vi "Attenuator Flatten Test Parameters.vi"(7 "Test Configuration (\"\")":string, 9 "error in (no error)":errorcluster, 10 "Parameter Variant":variant) -> (1 "error out":errorcluster, 2 "Parameter String":string)   [LabVIEW 2011]
uses:
  TypeDefs/Attenuator Test Parameters.ctl
  TypeDefs/Attenuator Stimulus Parameters.ctl
  TypeDefs/Attenuator ATT Stimulus.ctl
  TypeDefs/Attenuator VNA Stimulus.ctl
  S Parameter/TypeDefs/SP Frequency Units.ctl
  TypeDefs/Attenuator VNA Calibration State.ctl
  TypeDefs/Attenuator Measurement Cluster.ctl
  TypeDefs/Attenuator Limit.ctl
  TypeDefs/Attenuator Calibration State.ctl
  Attenuator Version.vi
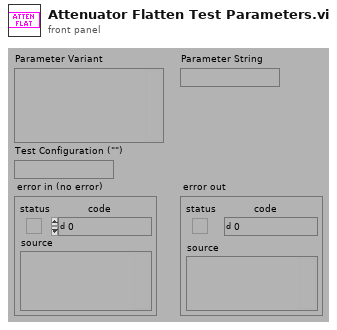
[diagram p1: front panel]
types:
  T1 = typedef "Attenuator Test Parameters.ctl" = cluster{"Stimulus":T2, "Measurement":T7, "Limit":T8, "Normalization":T9}
  T2 = typedef "Attenuator Stimulus Parameters.ctl" = cluster{"ATT Stimulus":T3, "VNA Stimulus":T4}
  T3 = typedef "Attenuator ATT Stimulus.ctl" = cluster{"Normalize":bool, "Value (dB)":dbl}
  T4 = typedef "Attenuator VNA Stimulus.ctl" = cluster{"Use Instrument Settings":bool, "Blank Frequencies":bool, "Sweep Type":enum32{"Linear", "Logarithmic", "List", "Power", "CW"}, "Sweep":cluster{"Fstart":dbl, "Fstop":dbl, "Units":T5, "Points":i32}, "Power (dBm)":dbl, "IFBW (Hz)":dbl, "Sweep Time (s)":dbl, "Calibration":T6}
  T5 = typedef "SP Frequency Units.ctl" = enum16{"Hz", "kHz", "MHz", "GHz", "Points"}
  T6 = typedef "Attenuator VNA Calibration State.ctl" = cluster{"State":bool, "String":string}
  T7 = typedef "Attenuator Measurement Cluster.ctl" = cluster{"Step (dB)":enum16{"0.25", "0.50", "1.00"}, "Start (dB)":dbl, "Stop (dB)":dbl}
  T8 = typedef "Attenuator Limit.ctl" = cluster{"Maximum Error":dbl}
  T9 = typedef "Attenuator Calibration State.ctl" = cluster{"Normalized?":bool, "Normalization Values (dB)":dbl[]}
  T10 = typedef "OGAB Version.ctl" = cluster{"Version":string, "Build Number":u32, "Build Date/Time":dbl}
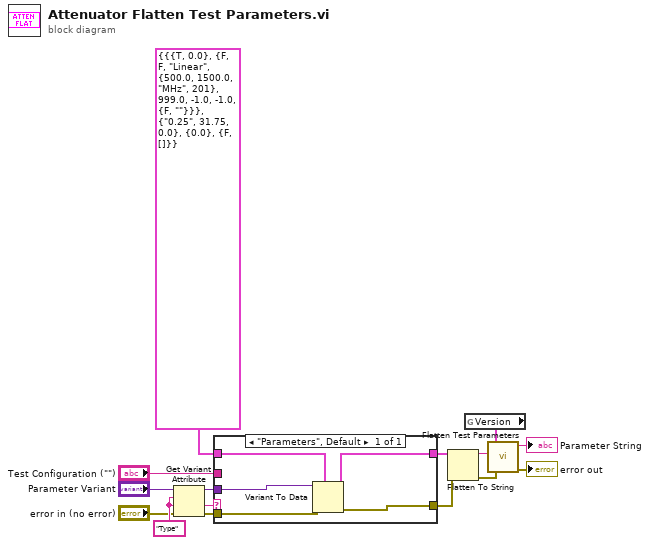
[diagram p0: block diagram]
diagram:
  w14 = "Type" ("name")
  n1 = Get Variant Attribute(Variant="Parameter Variant", name=w14, default value (empty Variant)=w14, error in="error in (no error)") -> (duplicate Variant=w4:variant, value=w3:string, error out=w7:errorcluster)  [unwired: 1 out]
  n2 = case shown="\"Parameters\", Default" w3 {
    tunnel: w4 -> [w20]
    tunnel: T1 {"Stimulus"={"ATT Stimulus"={"Normalize"=TRUE, "Value (dB)"=0.0}, "VNA Stimulus"={"Use Instrument Settings"=FALSE, "Blank Frequencies"=FALSE, "Sweep Type"=enum."Linear", "Sweep"={"Fstart"=500.0, "Fstop"=1500.0, "Units"=enum."MHz", "Points"=201}, "Power (dBm)"=999.0, "IFBW (Hz)"=-1.0, "Sweep Time (s)"=-1.0, "Calibration"={"State"=FALSE, "String"=""}}}, "Measurement"={"Step (dB)"=enum."0.25", "Start (dB)"=31.75, "Stop (dB)"=0.0}, "Limit"={"Maximum Error"=0.0}, "Normalization"={"Normalized?"=FALSE, "Normalization Values (dB)"=[]}} ("Attenuator Test Parameters") -> [w16]
    tunnel: [w17] -> w2
    tunnel: [w19] -> w5
    tunnel: w7 -> [w18]
    tunnel: "Test Configuration (\"\")" -> [_]
    frame "Parameters", Default {
      n3 = Variant To Data(error in=w18, type=w16, Variant=w20) -> (data=w17:T1, error out=w19:errorcluster)
    }
  }
  n4 = Flatten To String(anything=w2, error in (no error)=w5) -> (data string=w13:string, error out=w11:errorcluster)  [unwired: 3 out]
  n5 = global read "Attenuator Version.vi" "Version"() -> (w12:T10)
  n6 = call "Flatten Test Parameters.vi"("error in (no error)"=w11, "Flattened Test Parameters (\"\")"=w13, "Test Version"=w12) -> ("error out"=→"error out":errorcluster, "Flattened Test Parameters with Version"=→"Parameter String":string)  [unwired: 3 out]
